vi "HandleConfig.vi"(0 "Stand in":refnum<class "Stand.lvclass">, 11 "error in (no error)":errorcluster) -> (4 "Stand out":refnum<class "Stand.lvclass">, 15 "error out":errorcluster)   [LabVIEW 2019, in "Stand.lvclass"]
uses:
  Stand.lvclass
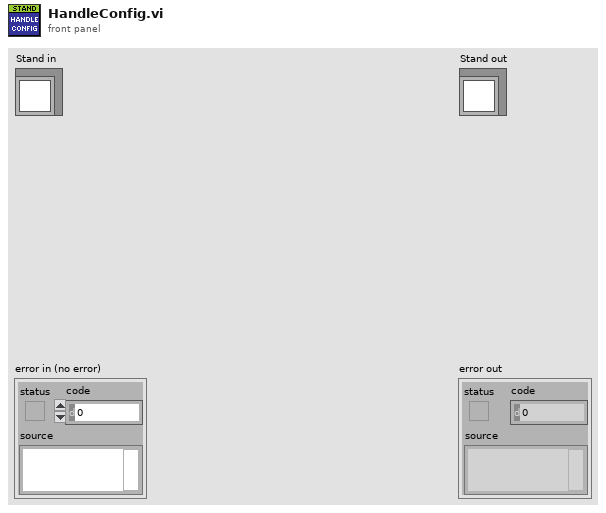
[diagram p1: front panel]
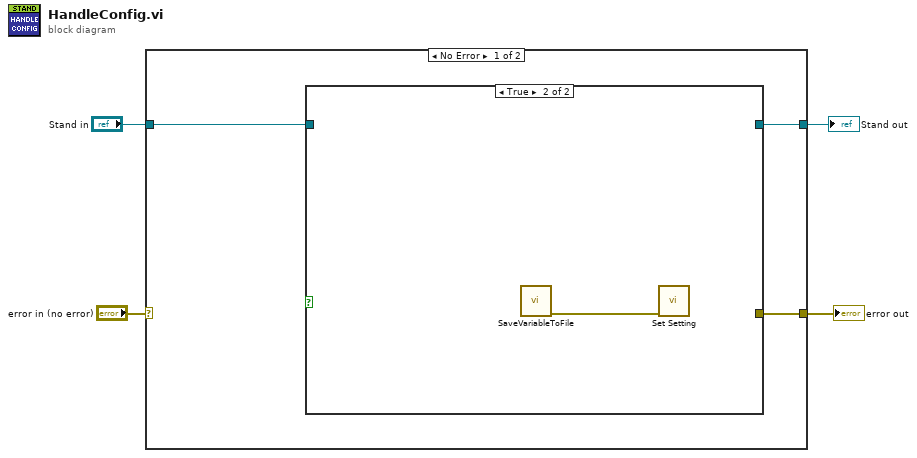
[diagram p0: block diagram]
diagram:
  n1 = case shown="No Error" "error in (no error)" {
    selector: "error in (no error)" -> [_ w12]
    tunnel: [w7 w12] -> w3
    tunnel: [w6 w11] -> w1
    tunnel: "Stand in" -> [w5 w11]
    frame No Error {
      n2 = case shown="True" {
        selector: _ -> [_ _]
        tunnel: [w8 _] -> w7
        tunnel: [w9 _] -> w6
        tunnel: w5 -> [w9 _]
        frame False {
        }
        frame True {
          n3 = call "SaveVariableToFile.vi"() -> ("error out"=w10:errorcluster)  [unwired: 15 in]
          n4 = call "Set Setting.vi"("error in (no error)"=w10) -> ()  [unwired: 9 in, 2 out]
        }
      }
    }
    frame Error {
    }
  }
  "error out" <- w3
  "Stand out" <- w1
